vi "Initialise - From List.vi"(6 "Tag Root":string, 8 "error in (no error)":errorcluster, 10 "Tag List":T1[](array[typedef]), 11 "Local Bus in":refnum<class "Local Bus.lvclass">) -> (0 "error out":errorcluster, 3 "Local Bus out":refnum<class "Local Bus.lvclass">)   [LabVIEW 2021, in "Local Bus.lvclass"]
uses:
  Local Bus.lvclass
  C:/Users/Tim/Documents/GitHub/Omni-Bus/Source/Omni-Bus/Bus Access/Bus_Access.lvclass
  Support/Tag List Type.ctl
  <vilib>/Utility/Data Type/Type Definitions/Data Type.ctl
  Omni-Bus/Bus Access/Bus_Access.lvclass/Bus_Access.ctl
  Local Bus.lvclass/Local Bus.ctl
  Omni-Bus/Bus Access/Properties/Write Tags.vi
  Properties/Write Tag Types.vi
  Omni-Bus/Bus Access/Properties/Write Tag Root.vi
  <vilib>/Utility/Data Type/NI_Data Type.lvlib
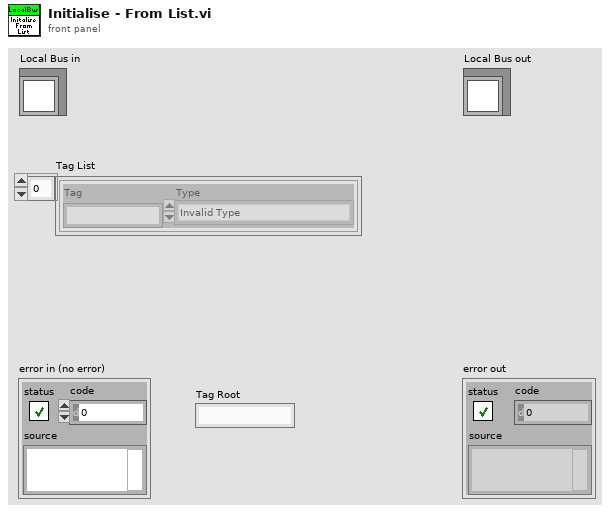
[diagram p1: front panel]
types:
  T1 = typedef "Local Bus.lvclass/Tag List Type.ctl" = cluster{"Tag":string, "Type":T2}
  T2 = typedef "NI_Data Type.lvlib/Data Type.ctl" = enum8{"Invalid Type", "Void", "I8", "I16", "I32", "I64", "U8", "U16", "U32", "U64", "Single Float", "Double Float", "Extended Float", "Single Complex", "Double Complex", "Extended Complex", "Enum U8", "Enum U16", "Enum U32", "Enum U64", "Single Float With Unit", "Double Float With Unit", "Extended Float With Unit", "Single Complex with Unit", "Double Complex with Unit", "Extended Complex with Unit", "Boolean", "String", "Path", "Picture", "Tag", "Array", "Cluster", "Variant", "LV Variant", "Waveform", "Timestamp", "Digital Waveform", "Digital Data", "ExpressData", "Refnum", "External Data", "VI", "Poly VI", "LabVIEW Class Instance", "Fixed Point", "Set Collection", "Map Collection"}
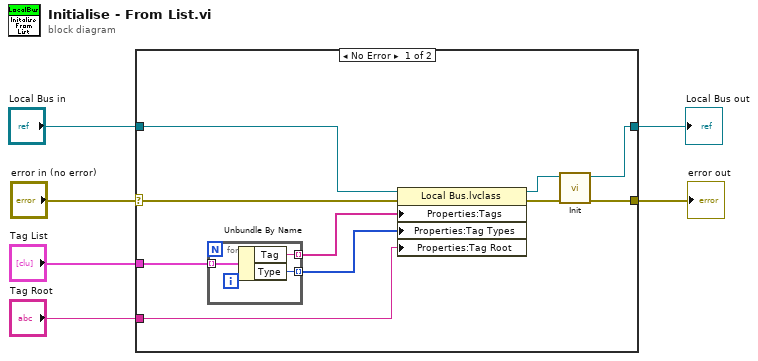
[diagram p0: block diagram]
diagram:
  n1 = case shown="No Error" "error in (no error)" {
    selector: "error in (no error)" -> [w16 w21]
    tunnel: [w9 w21] -> w5
    tunnel: [w7 w20] -> w3
    tunnel: "Local Bus in" -> [w15 w20]
    tunnel: "Tag List" -> [w14 _]
    tunnel: "Tag Root" -> [w11 _]
    frame No Error {
      n2 = for {
        tunnel: w14 -> [w19] mode=indexing
        tunnel: [w18] -> w13 mode=indexing
        tunnel: [w17] -> w12 mode=indexing
        n3 = Unbundle By Name(w19) -> ("Tag"=w18:string, "Type"=w17:T2)
      }
      n4 = property class="Local Bus.lvclass"(reference=w15, error in=w16, "Properties:Tags"=w13, "Properties:Tag Types"=w12, "Properties:Tag Root"=w11) -> (reference out=w8:refnum<class "Local Bus.lvclass">, error out=w10:errorcluster)
      n5 = call-dynamic "Init.vi"("error in (no error)"=w10, "Data in"=w8) -> ("error out"=w9:errorcluster, "Data out"=w7:refnum<class "Local Bus.lvclass">)  [unwired: 8 in]
    }
    frame Error {
    }
  }
  "error out" <- w5
  "Local Bus out" <- w3
